vi "Set MessageQ.vi"(10 "MessageQ":refnum<queue>, 11 "CD_Process in":refnum<class "CD_Process.lvclass">) -> (3 "CD_Process out":refnum<class "CD_Process.lvclass">)   [LabVIEW 2019, in "TimingDRV Engine.lvlib" / "CD_Process.lvclass"]
uses:
  CD_Process.lvclass
  TypeDefs/Message.ctl
  CD_Process.lvclass/CD_Process.ctl
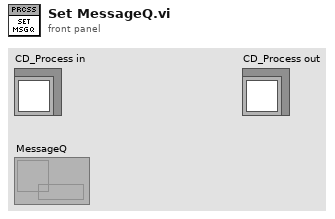
[diagram p1: front panel]
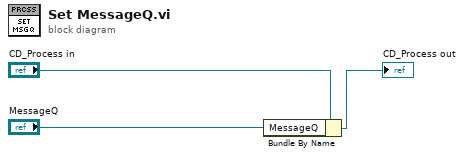
[diagram p0: block diagram]
diagram:
  n1 = Bundle By Name(cluster="CD_Process in", "MessageQ"="MessageQ") -> (→"CD_Process out":refnum<class "CD_Process.lvclass">)
